vi "sonictest 2.vi"   [LabVIEW 2010, in "Test1.lvrbt"]
uses:
  Test1.lvrbt
  <vilib>/NXT/Block Support/NXT_InputPort.ctl
  <vilib>/NXT/Subs/MotorOutput.ctl
  <vilib>/NXT/Dual Mode Library/Sensors/Sonar_cm.vi
  <vilib>/NXT/Dual Mode Library/Motors/MotorOn.vi
  <vilib>/NXT/Dual Mode Library/Motors/MotorBrake.vi
types:
  T1 = typedef "NXT_InputPort.ctl" = u8
  T2 = typedef "MotorOutput.ctl" = u8
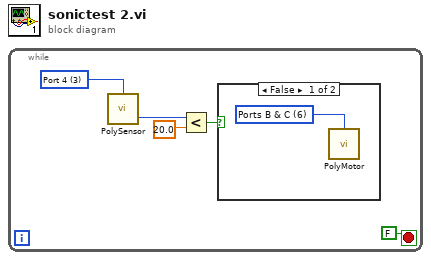
[diagram p0: block diagram]
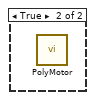
[diagram p2: hidden frame]
diagram:
  n1 = while {
    stop <- FALSE stop-if-true
    w1 = T1 3 items=["Port 1", "Port 2", "Port 3", "Port 4"] ("Port (Port 4)")
    n2 = call-poly <vilib>:"PolySensor.vi"("Port (Port 4)"=w1) -> ("Distance (cm)"=w5:i16)  [unwired: 2 in, 1 out]
    n3 = Less?(x=w5, y=20.0 ("x")) -> (x < y?=w3:bool)
    n4 = case shown="False" w3 {
      frame False {
        w6 = T2 6 items=["Port A"=0, "Port B"=1, "Port C"=2, "Ports A & B"=4, "Ports A & C"=5, "Ports B & C"=6, "All Ports"=3] ("Output Port (All Ports)")
        n5 = call-poly <vilib>:"PolyMotor.vi"("Output Port (All Ports)"=w6) -> ()  [unwired: 3 in, 1 out]
      }
      frame True {
        n6 = call-poly <vilib>:"PolyMotor.vi"() -> ()  [unwired: 4 in, 1 out]
      }
    }
  }
